vi "logfile-name.vi"() -> ()   [LabVIEW 2021]
panel:
  out "logfile_name":string="2020-07-25 home-F9P"
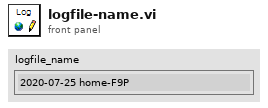
[diagram p1: front panel]
diagram:
